vi "FTW-Example-Endpoints.vi"() -> ()   [LabVIEW 2012]
uses:
  Actor/src/Utility/FTW-Actor-Address.ctl
  Actor/src/Utility/FTW-Actor-Configuration.ctl
  Actor/src/Endpoint/FTW-Endpoint.lvclass
  Actor/src/FTW-Actor.lvlib
  Actor/src/Ether/FTW-Ether.lvclass
panel:
  in  "Enpoint Type":enum32{"ZMQ-tcp", "ZMQ-inproc", "LabVIEW-lvq"}(radio)=enum."ZMQ-inproc"
  out "Timed out?":bool
  out "Actual Server Address":T1
  out "error out":errorcluster
  out "Response Body":string
  out "Response Header":string
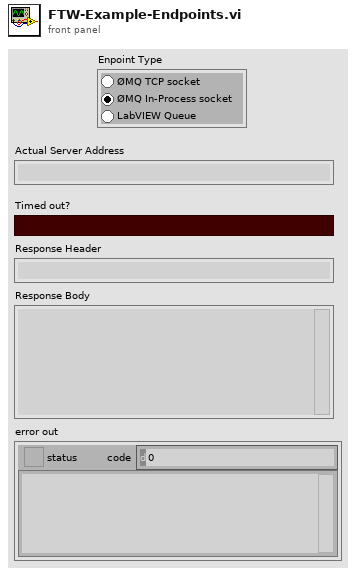
[diagram p1: front panel]
types:
  T1 = typedef "FTW-Actor.lvlib/FTW-Actor-Address.ctl" = string
  T2 = typedef "FTW-Actor.lvlib/FTW-Actor-Configuration.ctl" = string
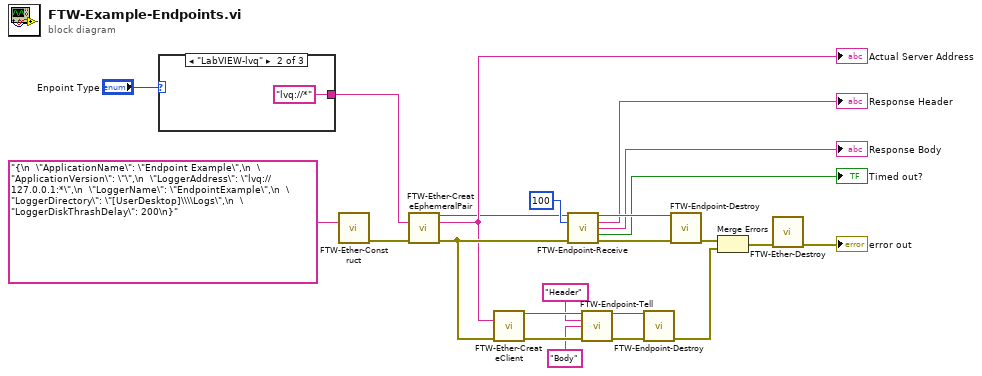
[diagram p0: block diagram]
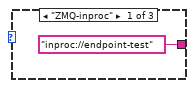
[diagram p2: hidden frame]
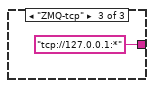
[diagram p3: hidden frame]
diagram:
  n1 = case shown="\"LabVIEW-lvq\"" "Enpoint Type" {
    tunnel: [T1 "inproc://endpoint-test" ("Server Address") T1 "lvq://*" ("Server Address") T1 "tcp://127.0.0.1:*" ("Server Address")] -> w1
    frame "ZMQ-inproc" {
    }
    frame "LabVIEW-lvq" {
    }
    frame "ZMQ-tcp" {
    }
  }
  n2 = call "FTW-Ether-Construct.vi"("FTW Ether Configuration"=T2 "{\n  \"ApplicationName\": \"Endpoint Example\",\n  \"ApplicationVersion\": \"\",\n  \"LoggerAddress\": \"lvq://127.0.0.1:*\",\n  \"LoggerName\": \"EndpointExample\",\n  \"LoggerDirectory\": \"[UserDesktop]\\\\Logs\",\n  \"LoggerDiskThrashDelay\": 200\n}") -> ("error out"=w6:errorcluster)  [unwired: 14 in]
  n3 = call "FTW-Ether-CreateEphemeralPair.vi"("Requested Ephemeral Address"=w1, "error in"=w6) -> ("Ephemeral Endpoint"=w3:refnum<class "FTW-Endpoint.lvclass">, "Actual Ephemeral Address"=w4:T1, "error out"=w5:errorcluster)  [unwired: 11 in]
  "Actual Server Address" <- w4
  n4 = call "FTW-Ether-CreateClient.vi"("Server Address"=w4, "error in"=w5) -> ("Client Endpoint"=w23:refnum<class "FTW-Endpoint.lvclass">, "error out"=w22:errorcluster)  [unwired: 12 in]
  n5 = call-dynamic "FTW-Endpoint-Receive.vi"("FTW Endpoint"=w3, "Timeout"=100, "error in"=w5) -> ("FTW Endpoint out"=w17:refnum<class "FTW-Endpoint.lvclass">, "Message Header"=→"Response Header":string, "Response Body"=→"Response Body":string, "Timed out?"=→"Timed out?":bool, "error out"=w16:errorcluster)  [unwired: 8 in]
  n6 = call-dynamic "FTW-Endpoint-Tell.vi"("FTW Endpoint"=w23, "Message Header"="Header", "Message Body"="Body", "error in"=w22) -> ("FTW Endpoint out"=w19:refnum<class "FTW-Endpoint.lvclass">, "error out"=w18:errorcluster)  [unwired: 9 in, 1 out]
  n7 = call-dynamic "FTW-Endpoint-Destroy.vi"("FTW Endpoint"=w19, "error in"=w18) -> ("error out"=w12:errorcluster)  [unwired: 13 in]
  n8 = call-dynamic "FTW-Endpoint-Destroy.vi"("FTW Endpoint"=w17, "error in"=w16) -> ("error out"=w13:errorcluster)  [unwired: 13 in]
  n9 = Merge Errors(w13, w12) -> (w11:errorcluster)
  n10 = call "FTW-Ether-Destroy.vi"("error in"=w11) -> ("error out"=→"error out":errorcluster)  [unwired: 14 in]
